vi "CoordSystem_Convert_Rotation3d.vi"(9 "CoordSys To":T1={"Rotation"={"Q_quaternion"={"R"=1.0, "V"=[0.0, 0.0, 0.0]}}}, 10 "CoordSys From":T1={"Rotation"={"Q_quaternion"={"R"=1.0, "V"=[0.0, 0.0, 0.0]}}}, 11 "in Rotation3d":T2={"Q_quaternion"={"R"=0.0, "V"=[0.0, 0.0, 0.0]}}) -> (3 "out Converted Rotation3d":T2)   [LabVIEW 2019, in "Trajectory_Library.lvlib"]
doc: "Converts the given rotation from one coordinate system to another.\n\nInputs:\n - in rotation3d -- The rotation to convert.\n - Coord Sys from -- The coordinate system the pose starts in.\n - Coord Sys to -- The coordinate system to which to convert.\n\nReturns:\n - Converted Rotation -- The given rotation in the desired coordinate system."
uses:
  Trajectory_Library.lvlib
  TypeDef/ROTATION3D.ctl
  TypeDef/QUATERNION.ctl
  TypeDef/COORDINATE_SYSTEM.ctl
  Rotation3d_UnaryMinus.vi
  Rotation3d_Create_Quaternion.vi
  Quaternion_Times.vi
  Rotation3d_GetQuaterion.vi
  Quaternion_Inverse.vi
  Quaternion_Normalize.vi
  Quaternion_New_Default.vi
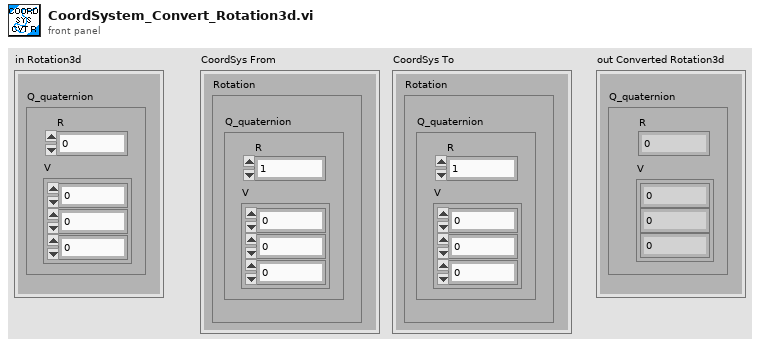
[diagram p1: front panel]
types:
  T1 = typedef "Trajectory_Library.lvlib/COORDINATE_SYSTEM.ctl" = cluster{"Rotation":T2}
  T2 = typedef "Trajectory_Library.lvlib/ROTATION3D.ctl" = cluster{"Q_quaternion":T3}
  T3 = typedef "Trajectory_Library.lvlib/QUATERNION.ctl" = cluster{"R":dbl, "V":dbl[]}
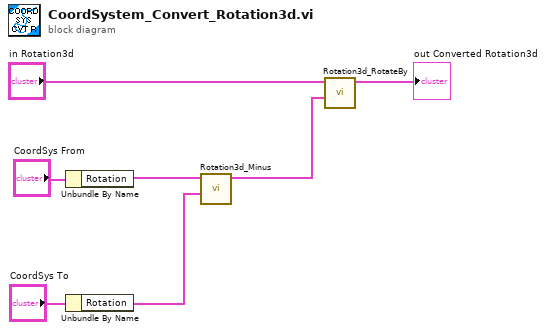
[diagram p0: block diagram]
diagram:
  n1 = Unbundle By Name("CoordSys From") -> ("Rotation"=w3:T2)
  n2 = Unbundle By Name("CoordSys To") -> ("Rotation"=w2:T2)
  n3 = call "Rotation3d_Minus.vi"("other Rotation3d"=w2, "in Rotation3d"=w3) -> ("out Rotation3d"=w1:T2)  [unwired: 9 in]
  n4 = call "Rotation3d_RotateBy.vi"("other Rotation3d"=w1, "in Rotation3d"="in Rotation3d") -> ("out Rotation3d"=→"out Converted Rotation3d":T2)  [unwired: 9 in]
